vi "Variant_Get_TS_Propss_LV2015.vi"(8 "error in (no error)":errorcluster, 9 "TS Paramter Ref Str":string="Step.Parameters", 10 "Sequence Context In":refnum<k7>, 11 "Variant (Type) In":variant) -> (0 "error out":errorcluster, 3 "Variant of Input Type":variant)   [LabVIEW 2015]
uses:
  <vilib>/addons/TestStand/_TSUtility.llb/TestStand - Get Property Value (Number {Signed 8-bit Integer}).vi
  <vilib>/addons/TestStand/_TSUtility.llb/TestStand - Get Property Value (Number {Signed 16-bit Integer}).vi
  <vilib>/addons/TestStand/_TSUtility.llb/TestStand - Get Property Value (Number {Signed 32-bit Integer}).vi
  <vilib>/addons/TestStand/_TSUtility.llb/TestStand - Get Property Value (Number {Signed 64-bit Integer}).vi
  <vilib>/addons/TestStand/_TSUtility.llb/TestStand - Get Property Value (Number {Unsigned 8-bit Integer}).vi
  <vilib>/addons/TestStand/_TSUtility.llb/TestStand - Get Property Value (Number {Unsigned 16-bit Integer}).vi
  <vilib>/addons/TestStand/_TSUtility.llb/TestStand - Get Property Value (Number {Unsigned 32-bit Integer}).vi
  <vilib>/addons/TestStand/_TSUtility.llb/TestStand - Get Property Value (Number {Unsigned 64-bit Integer}).vi
  <vilib>/addons/TestStand/_TSUtility.llb/TestStand - Get Property Value (Number).vi
  <vilib>/addons/TestStand/_TSUtility.llb/TestStand - Get Property Value (Boolean).vi
  <vilib>/addons/TestStand/_TSUtility.llb/TestStand - Get Property Value (String).vi
  <vilib>/addons/TestStand/_TSUtility.llb/TestStand - Get Property Value (Reference).vi
panel:
  # "Connector Pane"
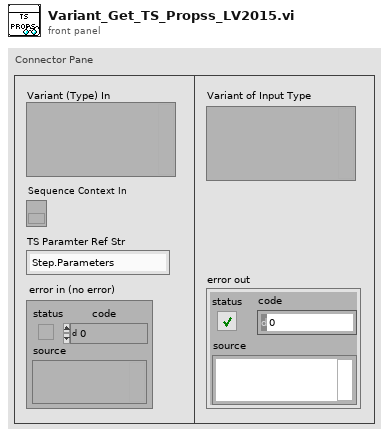
[diagram p1: front panel]
types:
  T1 = typedef "Type Descriptor Enumeration__ogtk.ctl" = enum8{"<Null>", "I8", "I16", "I32", "I64", "U8", "U16", "U32", "U64", "SGL", "DBL", "EXT", "CSG", "CDB", "CXT", "0x0F", "0x10", "0x11", "0x12", "0x13", "0x14", "Enum U8", "Enum U16", "Enum U32", "Enum U64", "SGL PQ", "DBL PQ", "EXT PQ", "CSG PQ", "CDB PQ", "CXT PQ", "0x1F", "0x20", "Boolean", "0x22", "0x23", "0x24", "0x25", "0x26", "0x27", "0x28", "0x29", "0x2A", "0x2B", "0x2C", "0x2D", "0x2E", "0x2F", "String", "0x31", "Path", "Pict", "0x34", "0x35", "0x36", "DAQ", "0x38", "0x39", "0x3A", "0x3B", "0x3C", "0x3D", "0x3E", "0x3F", "Array", "0x41", "0x42", "0x43", "0x44", "0x45", "0x46", "0x47", "0x48", "0x49", "0x4A", "0x4B", "0x4C", "0x4D", "0x4E", "0x4F", "Cluster", "0x51", "0x52", "Variant", "Waveform", "0x55", "0x56", "0x57", "0x58", "0x59", "0x5A", "0x5B", "0x5C", "0x5D", "0x5E", "0x5F", "0x60", "0x61", "0x62", "0x63", "0x64", "0x65", "0x66", "0x67", "0x68", "0x69", "0x6A", "0x6B", "0x6C", "0x6D", "0x6E", "0x6F", "Refnum"}
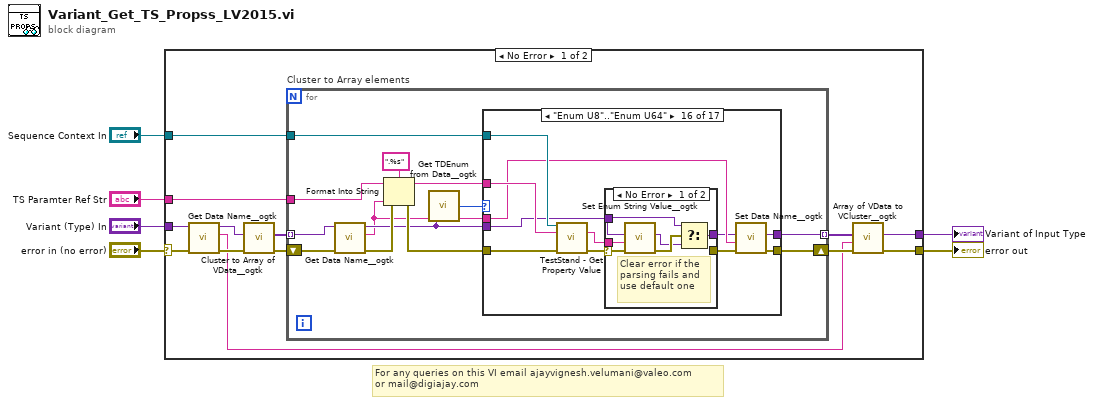
[diagram p0: block diagram]
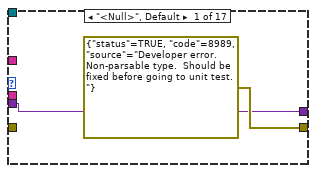
[diagram p2: hidden frame]
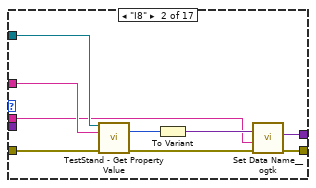
[diagram p3: hidden frame]
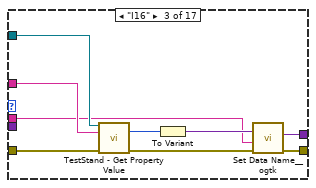
[diagram p4: hidden frame]
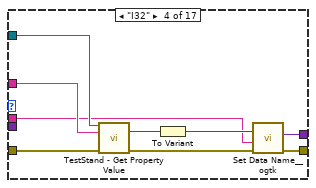
[diagram p5: hidden frame]
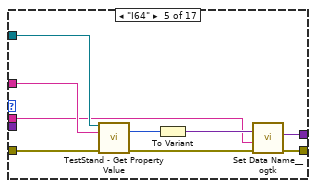
[diagram p6: hidden frame]
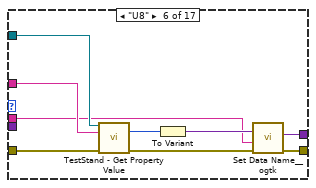
[diagram p7: hidden frame]
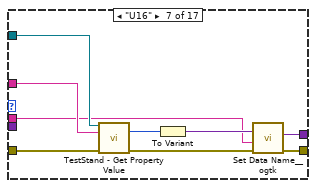
[diagram p8: hidden frame]
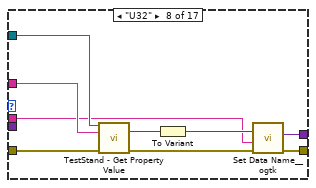
[diagram p9: hidden frame]
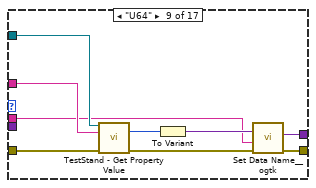
[diagram p10: hidden frame]
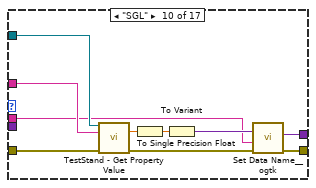
[diagram p11: hidden frame]
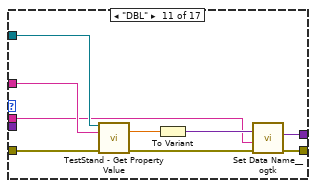
[diagram p12: hidden frame]
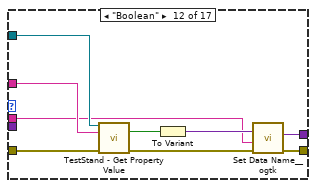
[diagram p13: hidden frame]
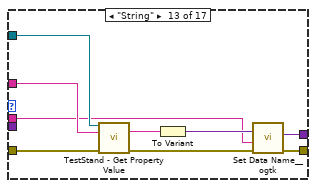
[diagram p14: hidden frame]
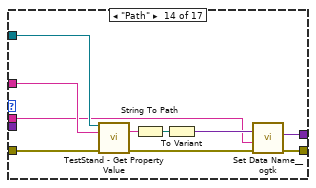
[diagram p15: hidden frame]
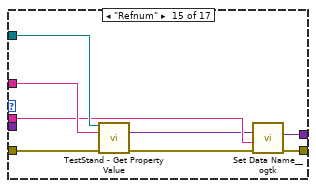
[diagram p16: hidden frame]
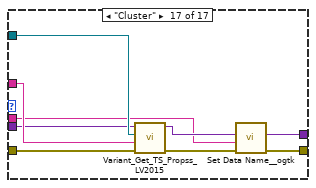
[diagram p18: hidden frame]
diagram:
  # "For any queries on this VI email ajayvignesh.velumani@valeo.com\nor mail@digiajay.com"
  n1 = case shown="No Error" "error in (no error)" {
    selector: "error in (no error)" -> [w11 w191]
    tunnel: "TS Paramter Ref Str" -> [w16 _]
    tunnel: "Sequence Context In" -> [w15 _]
    tunnel: [w14 w191] -> w4
    tunnel: [w12 w190] -> w3
    tunnel: "Variant (Type) In" -> [w9 w190]
    frame No Error {
      n2 = call <userlib>:"Get Data Name__ogtk.vi"("error in (no error)"=w11, "Data"=w9) -> ("error out"=w10:errorcluster, "Data Name"=w7:string, "Data dup"=w8:variant)  [unwired: 7 in]
      n3 = call <userlib>:"Cluster to Array of VData__ogtk.vi"("error in (no error)"=w10, "Cluster"=w8) -> ("error out"=w18:errorcluster, "Array of VData"=w19:variant[])  [unwired: 8 in]
      n4 = for "Cluster to Array elements" {
        tunnel: w19 -> [w32] mode=indexing
        shift-right: [w30] -> w17
        shift-left: w18 -> [w31]
        tunnel: w16 -> [w25]
        tunnel: w15 -> [w23]
        tunnel: [w20] -> w13 mode=indexing
        n5 = call <userlib>:"Get Data Name__ogtk.vi"("error in (no error)"=w31, "Data"=w32) -> ("error out"=w28:errorcluster, "Data Name"=w21:string, "Data dup"=w22:variant)  [unwired: 7 in]
        n6 = Format Into String(format string=".%s", initial string=w25, error in=w28, w21) -> (resulting string=w24:string, error out=w27:errorcluster)
        n7 = call <userlib>:"Get TDEnum from Data__ogtk.vi"("Data"=w22) -> ("Type Descriptor Enumeration"=w29:T1)  [unwired: 4 in]
        n8 = case shown="\"Enum U8\"..\"Enum U64\"" w29 {
          tunnel: [errorcluster {"status"=TRUE, "code"=8989, "source"="Developer error.  Non-parsable type.  Should be fixed before going to unit test."} ("error out") w38 w47 w56 w65 w74 w83 w92 w101 w111 w120 w129 w138 w148 w157 w168 w184] -> w30
          tunnel: w27 -> [_ w42 w51 w60 w69 w78 w87 w96 w105 w115 w124 w133 w142 w152 w160 w169 w189]
          tunnel: w24 -> [_ w41 w50 w59 w68 w77 w86 w95 w104 w114 w123 w132 w141 w151 w159 w171 w187]
          tunnel: w22 -> [w33 _ _ _ _ _ _ _ _ _ _ _ _ _ _ w164 w185]
          tunnel: w23 -> [_ w40 w49 w58 w67 w76 w85 w94 w103 w113 w122 w131 w140 w150 w158 w170 w186]
          tunnel: w21 -> [_ w36 w45 w54 w63 w72 w81 w90 w99 w109 w118 w127 w136 w146 w156 w166 w181]
          tunnel: [w33 w35 w44 w53 w62 w71 w80 w89 w98 w108 w117 w126 w135 w145 w155 w167 w182] -> w20
          frame "<Null>", Default {
          }
          frame "I8" {
            n9 = call-poly <vilib>:"TestStand - Get Property Value.vi"("Sequence Context In"=w40, "Lookup String"=w41, "error in (no error)"=w42) -> ("Value"=w39:i8, "error out"=w43:errorcluster)  [unwired: 10 in, 1 out]
            n10 = To Variant(anything=w39) -> (Variant=w37:variant)
            n11 = call <userlib>:"Set Data Name__ogtk.vi"("error in (no error)"=w43, "Data Name"=w36, "Data"=w37) -> ("error out"=w38:errorcluster, "Renamed Data"=w35:variant)  [unwired: 7 in]
          }
          frame "I16" {
            n12 = call-poly <vilib>:"TestStand - Get Property Value.vi"("Sequence Context In"=w49, "Lookup String"=w50, "error in (no error)"=w51) -> ("Value"=w48:i16, "error out"=w52:errorcluster)  [unwired: 10 in, 1 out]
            n13 = To Variant(anything=w48) -> (Variant=w46:variant)
            n14 = call <userlib>:"Set Data Name__ogtk.vi"("error in (no error)"=w52, "Data Name"=w45, "Data"=w46) -> ("error out"=w47:errorcluster, "Renamed Data"=w44:variant)  [unwired: 7 in]
          }
          frame "I32" {
            n15 = call-poly <vilib>:"TestStand - Get Property Value.vi"("Sequence Context In"=w58, "Lookup String"=w59, "error in (no error)"=w60) -> ("Value"=w57:i32, "error out"=w61:errorcluster)  [unwired: 10 in, 1 out]
            n16 = To Variant(anything=w57) -> (Variant=w55:variant)
            n17 = call <userlib>:"Set Data Name__ogtk.vi"("error in (no error)"=w61, "Data Name"=w54, "Data"=w55) -> ("error out"=w56:errorcluster, "Renamed Data"=w53:variant)  [unwired: 7 in]
          }
          frame "I64" {
            n18 = call-poly <vilib>:"TestStand - Get Property Value.vi"("Sequence Context In"=w67, "Lookup String"=w68, "error in (no error)"=w69) -> ("Value"=w66:i64, "error out"=w70:errorcluster)  [unwired: 10 in, 1 out]
            n19 = To Variant(anything=w66) -> (Variant=w64:variant)
            n20 = call <userlib>:"Set Data Name__ogtk.vi"("error in (no error)"=w70, "Data Name"=w63, "Data"=w64) -> ("error out"=w65:errorcluster, "Renamed Data"=w62:variant)  [unwired: 7 in]
          }
          frame "U8" {
            n21 = call-poly <vilib>:"TestStand - Get Property Value.vi"("Sequence Context In"=w76, "Lookup String"=w77, "error in (no error)"=w78) -> ("Value"=w75:u8, "error out"=w79:errorcluster)  [unwired: 10 in, 1 out]
            n22 = To Variant(anything=w75) -> (Variant=w73:variant)
            n23 = call <userlib>:"Set Data Name__ogtk.vi"("error in (no error)"=w79, "Data Name"=w72, "Data"=w73) -> ("error out"=w74:errorcluster, "Renamed Data"=w71:variant)  [unwired: 7 in]
          }
          frame "U16" {
            n24 = call-poly <vilib>:"TestStand - Get Property Value.vi"("Sequence Context In"=w85, "Lookup String"=w86, "error in (no error)"=w87) -> ("Value"=w84:u16, "error out"=w88:errorcluster)  [unwired: 10 in, 1 out]
            n25 = To Variant(anything=w84) -> (Variant=w82:variant)
            n26 = call <userlib>:"Set Data Name__ogtk.vi"("error in (no error)"=w88, "Data Name"=w81, "Data"=w82) -> ("error out"=w83:errorcluster, "Renamed Data"=w80:variant)  [unwired: 7 in]
          }
          frame "U32" {
            n27 = call-poly <vilib>:"TestStand - Get Property Value.vi"("Sequence Context In"=w94, "Lookup String"=w95, "error in (no error)"=w96) -> ("Value"=w93:u32, "error out"=w97:errorcluster)  [unwired: 10 in, 1 out]
            n28 = To Variant(anything=w93) -> (Variant=w91:variant)
            n29 = call <userlib>:"Set Data Name__ogtk.vi"("error in (no error)"=w97, "Data Name"=w90, "Data"=w91) -> ("error out"=w92:errorcluster, "Renamed Data"=w89:variant)  [unwired: 7 in]
          }
          frame "U64" {
            n30 = call-poly <vilib>:"TestStand - Get Property Value.vi"("Sequence Context In"=w103, "Lookup String"=w104, "error in (no error)"=w105) -> ("Value"=w102:u64, "error out"=w106:errorcluster)  [unwired: 10 in, 1 out]
            n31 = To Variant(anything=w102) -> (Variant=w100:variant)
            n32 = call <userlib>:"Set Data Name__ogtk.vi"("error in (no error)"=w106, "Data Name"=w99, "Data"=w100) -> ("error out"=w101:errorcluster, "Renamed Data"=w98:variant)  [unwired: 7 in]
          }
          frame "SGL" {
            n33 = call-poly <vilib>:"TestStand - Get Property Value.vi"("Sequence Context In"=w113, "Lookup String"=w114, "error in (no error)"=w115) -> ("Value"=w112:dbl, "error out"=w116:errorcluster)  [unwired: 10 in, 1 out]
            n34 = To Single Precision Float(number=w112) -> (single precision float=w107:sgl)
            n35 = To Variant(anything=w107) -> (Variant=w110:variant)
            n36 = call <userlib>:"Set Data Name__ogtk.vi"("error in (no error)"=w116, "Data Name"=w109, "Data"=w110) -> ("error out"=w111:errorcluster, "Renamed Data"=w108:variant)  [unwired: 7 in]
          }
          frame "DBL" {
            n37 = call-poly <vilib>:"TestStand - Get Property Value.vi"("Sequence Context In"=w122, "Lookup String"=w123, "error in (no error)"=w124) -> ("Value"=w121:dbl, "error out"=w125:errorcluster)  [unwired: 10 in, 1 out]
            n38 = To Variant(anything=w121) -> (Variant=w119:variant)
            n39 = call <userlib>:"Set Data Name__ogtk.vi"("error in (no error)"=w125, "Data Name"=w118, "Data"=w119) -> ("error out"=w120:errorcluster, "Renamed Data"=w117:variant)  [unwired: 7 in]
          }
          frame "Boolean" {
            n40 = call-poly <vilib>:"TestStand - Get Property Value.vi"("Sequence Context In"=w131, "Lookup String"=w132, "error in (no error)"=w133) -> ("Value"=w130:bool, "error out"=w134:errorcluster)  [unwired: 10 in, 1 out]
            n41 = To Variant(anything=w130) -> (Variant=w128:variant)
            n42 = call <userlib>:"Set Data Name__ogtk.vi"("error in (no error)"=w134, "Data Name"=w127, "Data"=w128) -> ("error out"=w129:errorcluster, "Renamed Data"=w126:variant)  [unwired: 7 in]
          }
          frame "String" {
            n43 = call-poly <vilib>:"TestStand - Get Property Value.vi"("Sequence Context In"=w140, "Lookup String"=w141, "error in (no error)"=w142) -> ("Value"=w139:string, "error out"=w143:errorcluster)  [unwired: 10 in, 1 out]
            n44 = To Variant(anything=w139) -> (Variant=w137:variant)
            n45 = call <userlib>:"Set Data Name__ogtk.vi"("error in (no error)"=w143, "Data Name"=w136, "Data"=w137) -> ("error out"=w138:errorcluster, "Renamed Data"=w135:variant)  [unwired: 7 in]
          }
          frame "Path" {
            n46 = call-poly <vilib>:"TestStand - Get Property Value.vi"("Sequence Context In"=w150, "Lookup String"=w151, "error in (no error)"=w152) -> ("Value"=w149:string, "error out"=w153:errorcluster)  [unwired: 10 in, 1 out]
            n47 = String To Path(string=w149) -> (path=w144:path)
            n48 = To Variant(anything=w144) -> (Variant=w147:variant)
            n49 = call <userlib>:"Set Data Name__ogtk.vi"("error in (no error)"=w153, "Data Name"=w146, "Data"=w147) -> ("error out"=w148:errorcluster, "Renamed Data"=w145:variant)  [unwired: 7 in]
          }
          frame "Refnum" {
            n50 = call-poly <vilib>:"TestStand - Get Property Value.vi"("Sequence Context In"=w158, "Lookup String"=w159, "error in (no error)"=w160) -> ("Value"=w154:variant, "error out"=w161:errorcluster)  [unwired: 10 in, 1 out]
            n51 = call <userlib>:"Set Data Name__ogtk.vi"("error in (no error)"=w161, "Data Name"=w156, "Data"=w154) -> ("error out"=w157:errorcluster, "Renamed Data"=w155:variant)  [unwired: 7 in]
          }
          frame "Enum U8".."Enum U64" {
            n52 = call-poly <vilib>:"TestStand - Get Property Value.vi"("Sequence Context In"=w170, "Lookup String"=w171, "error in (no error)"=w169) -> ("Value"=w165:string, "error out"=w172:errorcluster)  [unwired: 10 in, 1 out]
            n53 = case shown="No Error" w172 {
              selector: w172 -> [w178 w180]
              tunnel: w165 -> [w177 _]
              tunnel: w164 -> [w175 w179]
              tunnel: [w173 w179] -> w163
              tunnel: [_ w180] -> w162
              frame No Error {
                # "Clear error if the\nparsing fails and \nuse default one"
                n54 = call <userlib>:"Set Enum String Value__ogtk.vi"("error in (no error)"=w178, "String Value"=w177, "Default Enum Value"=w175) -> ("error out"=w176:errorcluster, "Enum"=w174:variant)  [unwired: 7 in]
                n55 = Select(t=w175, s=w176, f=w174) -> (s? t:f=w173:variant)
              }
              frame Error {
              }
            }
            n56 = call <userlib>:"Set Data Name__ogtk.vi"("error in (no error)"=w162, "Data Name"=w166, "Data"=w163) -> ("error out"=w168:errorcluster, "Renamed Data"=w167:variant)  [unwired: 7 in]
          }
          frame "Cluster" {
            n57 = call "Variant_Get_TS_Propss_LV2015.vi"("error in (no error)"=w189, "TS Paramter Ref Str"=w187, "Sequence Context In"=w186, "Variant (Type) In"=w185) -> ("error out"=w188:errorcluster, "Variant of Input Type"=w183:variant)  [unwired: 6 in]
            n58 = call <userlib>:"Set Data Name__ogtk.vi"("error in (no error)"=w188, "Data Name"=w181, "Data"=w183) -> ("error out"=w184:errorcluster, "Renamed Data"=w182:variant)  [unwired: 7 in]
          }
        }
      }
      n59 = call <userlib>:"Array of VData to VCluster__ogtk.vi"("error in (no error)"=w17, "Cluster Name"=w7, "Array"=w13) -> ("error out"=w14:errorcluster, "VCluster"=w12:variant)  [unwired: 7 in]
    }
    frame Error {
    }
  }
  "error out" <- w4
  "Variant of Input Type" <- w3
